vi "诊断标定3 - 副本.vi"(8 "CAN端口":u16(ring), 9 "设备索引号":u16(ring), 10 "CAN卡类型":u32(ring)=21) -> ()   [LabVIEW 2013] (continued)
                    }
                    frame True {
                      n418 = case shown="假" w611 {
                        tunnel: w618 -> [w622 _]
                        tunnel: w617 -> [w621 _]
                        tunnel: w616 -> [w620 _]
                        tunnel: w612 -> [w619 w846]
                        frame False {
                          n419 = case shown="89" w620 {
                            tunnel: w621 -> [_ w625]
                            tunnel: w622 -> [_ w624]
                            tunnel: w619 -> [_ _]
                            frame 0, Default {
                            }
                            frame 137 {
                              n420 = case shown="1" w625 {
                                tunnel: w624 -> [_ w653 w697 w717 w844]
                                frame 0, Default {
                                }
                                frame 1 {
                                w635 = "." ("字符串")
                                n421 = Array Subset(array=w653, index=0 ("索引"), length=14 ("长度")) -> (w666:u8[])
                                n422 = Index Array(array=w653, index=14 ("索引")) -> (element=w656:u8)
                                n423 = Index Array(array=w653, index #1=15 ("索引"), index #2=16 ("索引")) -> (element #1=w662:u8, element #2=w663:u8)
                                n424 = Index Array(array=w653, index #1=17 ("索引"), index #2=18 ("索引")) -> (element #1=w657:u8, element #2=w658:u8)
                                n425 = call "数组去零.vi"("输入"=w666) -> ("输出"=w641:dbl[])
                                n426 = Join Numbers(hi=w657, lo=w658) -> ((hi.lo)=w654:u16)
                                n427 = Join Numbers(hi=w662, lo=w663) -> ((hi.lo)=w655:u16)
                                n428 = Number To Decimal String(number=w656) -> (decimal integer string=w648:string)  [unwired: 1 out]
                                n429 = Byte Array To String(unsigned byte array=w641) -> (string=w640:string)
                                n430 = Number To Decimal String(number=w654) -> (decimal integer string=w636:string)  [unwired: 1 out]
                                n431 = Number To Decimal String(number=w655) -> (decimal integer string=w647:string)  [unwired: 1 out]
                                n432 = Array Subset(array=w653, index=21 ("索引"), length=7 ("长度")) -> (w650:u8[])
                                n433 = Concatenate Strings("V" ("字符串"), w648, w635, w647, w635, w636) -> (w645:string)
                                n434 = call "数组去零.vi"("输入"=w650) -> ("输出"=w633:dbl[])
                                n435 = Byte Array To String(unsigned byte array=w633) -> (string=w631:string)
                                n436 = call <vilib>:"Space Constant.vi"() -> ("String"=w632:string)
                                n437 = Equal?(x=w631, y=w632) -> (x = y?=w637:bool)
                                n438 = Concatenate Strings("-" ("字符串"), w631) -> (w638:string)
                                n439 = Select(t=w632, s=w637, f=w638) -> (s? t:f=w634:string)
                                n440 = Concatenate Strings(w640, "-" ("字符串"), w645, w634) -> (w627:string)
                                n441 = local read "项目软件版本"() -> (w629:string[])
                                n442 = local read "从板板号"() -> (w626:u8)
                                n443 = local write "项目软件版本号"(w627) -> ()
                                n444 = Replace Array Subset(array=w629, new element=w627, index=w626) -> (w628:string[])
                                n445 = control-ref of="结果"() -> (w644:refnum<vi>)
                                n446 = local write "项目软件版本"(w628) -> ()
                                n447 = Build Array("项目软件版本     读取完成" ("读取结果")) -> (w642:string[])
                                n448 = call "表格编辑(版本读取).vi"("新元素/子数组"=w642, "活动单元格:单元格背景色"=u32 6618880, "MCListbox引用句柄"=w644) -> ()  [unwired: 9 out]
                                }
                                frame 2 {
                                w680 = ""
                                w677 = "." ("字符串")
                                n449 = Array Subset(array=w697, index=0 ("索引"), length=14 ("长度")) -> (w685:u8[])
                                n450 = Index Array(array=w697, index=14 ("索引")) -> (element=w700:u8)
                                n451 = Index Array(array=w697, index #1=15 ("索引"), index #2=16 ("索引")) -> (element #1=w706:u8, element #2=w707:u8)
                                n452 = Index Array(array=w697, index #1=17 ("索引"), index #2=18 ("索引")) -> (element #1=w701:u8, element #2=w702:u8)
                                n453 = Join Numbers(hi=w701, lo=w702) -> ((hi.lo)=w698:u16)
                                n454 = Join Numbers(hi=w706, lo=w707) -> ((hi.lo)=w699:u16)
                                n455 = Number To Decimal String(number=w698) -> (decimal integer string=w678:string)  [unwired: 1 out]
                                n456 = call "数组去零.vi"("输入"=w685) -> ("输出"=w684:dbl[])
                                n457 = Number To Decimal String(number=w700) -> (decimal integer string=w692:string)  [unwired: 1 out]
                                n458 = Number To Decimal String(number=w699) -> (decimal integer string=w691:string)  [unwired: 1 out]
                                n459 = Array Subset(array=w697, index=21 ("索引"), length=7 ("长度")) -> (w694:u8[])
                                n460 = Byte Array To String(unsigned byte array=w684) -> (string=w679:string)
                                n461 = call "数组去零.vi"("输入"=w694) -> ("输出"=w676:dbl[])
                                n462 = Concatenate Strings("V" ("字符串"), w692, w677, w691, w677, w678) -> (w689:string)
                                n463 = Byte Array To String(unsigned byte array=w676) -> (string=w674:string)
                                n464 = Equal?(x=w680, y=w674) -> (x = y?=w681:bool)
                                n465 = Concatenate Strings("-" ("字符串"), w674) -> (w682:string)
                                n466 = Select(t=w680, s=w681, f=w682) -> (s? t:f=w675:string)
                                n467 = Concatenate Strings(w679, "-" ("字符串"), w689, w675) -> (w670:string)
                                n468 = local read "平台软件版本"() -> (w672:string[])
                                n469 = local read "从板板号"() -> (w669:u8)
                                n470 = local write "平台软件版本号"(w670) -> ()
                                n471 = Replace Array Subset(array=w672, new element=w670, index=w669) -> (w671:string[])
                                n472 = control-ref of="结果"() -> (w687:refnum<vi>)
                                n473 = local write "平台软件版本"(w671) -> ()
                                n474 = Build Array("平台软件版本     读取完成" ("读取结果")) -> (w686:string[])
                                n475 = call "表格编辑(版本读取).vi"("新元素/子数组"=w686, "活动单元格:单元格背景色"=u32 6618880, "MCListbox引用句柄"=w687) -> ()  [unwired: 1 in, 8 out]
                                }
                                frame 3 {
                                n476 = Index Array(array=w717, index #1=0 ("索引"), index #2=1 ("索引")) -> (element #1=w713:u8, element #2=w714:u8)
                                n477 = Join Numbers(hi=w713, lo=w714) -> ((hi.lo)=w712:u16)
                                n478 = case shown="99, 默认" w712 {
                                tunnel: w717 -> [w720 _ w754]
                                tunnel: w712 -> [_ _ w732]
                                frame 0 {
                                n479 = Index Array(array=w720, index #1=2 ("索引"), index #2=3 ("索引")) -> (element #1=w724:u8, element #2=w723:u8)
                                n480 = Join Numbers(hi=w724, lo=w723) -> ((hi.lo)=w719:u16)
                                n481 = for {
                                N: w719 -> [_]
                                tunnel: w720 -> [w729]
                                tunnel: [w725] -> w718 mode=indexing
                                i -> [w728]
                                n482 = Add(x=w728, y=4) -> (x+y=w726:i32)
                                n483 = Index Array(array=w729, index=w726) -> (element=w725:u8)
                                }
                                "MODEL号" <- w718
                                }
                                frame 99, Default {
                                }
                                frame 1..40 {
                                w737 = ""
                                w758 = "." ("字符串")
                                n484 = Array Subset(array=w754, index=2 ("索引"), length=14 ("长度")) -> (w743:u8[])
                                n485 = Index Array(array=w754, index=16 ("索引")) -> (element=w766:u8)
                                n486 = Index Array(array=w754, index #1=17 ("索引"), index #2=18 ("索引")) -> (element #1=w772:u8, element #2=w773:u8)
                                n487 = Index Array(array=w754, index #1=19 ("索引"), index #2=20 ("索引")) -> (element #1=w767:u8, element #2=w768:u8)
                                n488 = Join Numbers(hi=w767, lo=w768) -> ((hi.lo)=w764:u16)
                                n489 = Join Numbers(hi=w772, lo=w773) -> ((hi.lo)=w765:u16)
                                n490 = Number To Decimal String(number=w732) -> (decimal integer string=w752:string)  [unwired: 1 out]
                                n491 = Number To Decimal String(number=w766) -> (decimal integer string=w760:string)  [unwired: 1 out]
                                n492 = call "数组去零.vi"("输入"=w743) -> ("输出"=w742:dbl[])
                                n493 = Number To Decimal String(number=w765) -> (decimal integer string=w759:string)  [unwired: 1 out]
                                n494 = Number To Decimal String(number=w764) -> (decimal integer string=w757:string)  [unwired: 1 out]
                                n495 = Byte Array To String(unsigned byte array=w742) -> (string=w744:string)
                                n496 = Concatenate Strings("第" ("读取结果"), w752, "模块" ("字符串"), "     读取完成" ("读取结果")) -> (w745:string)
                                n497 = Concatenate Strings("V" ("字符串"), w760, w758, w759, w758, w757) -> (w755:string)
                                n498 = control-ref of="结果"() -> (w748:refnum<vi>)
                                n499 = Array Subset(array=w754, index=23 ("索引"), length=7 ("长度")) -> (w741:u8[])
                                n500 = call "数组去零.vi"("输入"=w741) -> ("输出"=w736:dbl[])
                                n501 = Byte Array To String(unsigned byte array=w736) -> (string=w733:string)
                                n502 = Build Array(w745) -> (w747:string[])
                                n503 = control-ref of="模块软件版本 2"() -> (w749:refnum<vi>)
                                n504 = local read "模块软件版本"() -> (w750:T1)
                                n505 = Equal?(x=w737, y=w733) -> (x = y?=w738:bool)
                                n506 = call "表格编辑(版本读取).vi"("新元素/子数组"=w747, "活动单元格:单元格背景色"=u32 6618880, "MCListbox引用句柄"=w748) -> ()  [unwired: 1 in, 8 out]
                                n507 = Concatenate Strings("-" ("字符串"), w733) -> (w739:string)
                                n508 = Select(t=w737, s=w738, f=w739) -> (s? t:f=w735:string)
                                n509 = Concatenate Strings(w744, "-" ("字符串"), w755, w735) -> (w734:string)
                                n510 = case shown="30" w732 {
                                tunnel: [_ "VERSIONM" "BCUMCAL" "BMUMCAL" "BMURMCAL" "BCUCMCAL" "BCUDMCAL" "SCH" "BSW" "CDD" "DATALAYER" "DATAANALYSIS" "SOC" "SOH" "SOF" "INTRES" "INTCAN" "CARCAN" "CHGCANL" "THM" "CHGM" "HVM" "LVM" "BALM" "SAFEM" "RUNMODEM" "RELAY" "DO" "GBCHGDET" "SUPPLYPOWGDET" "SUMVDET" "CURDET" "TEMPERDET" "CELLVDET" "ISODET" "AI" "DI" "SYSCONF" "ECUCONF"] -> w731
                                frame 0, Default {
                                }
                                frame 1 {
                                }
                                frame 2 {
                                }
                                frame 3 {
                                }
                                frame 4 {
                                }
                                frame 5 {
                                }
                                frame 6 {
                                }
                                frame 7 {
                                }
                                frame 8 {
                                }
                                frame 9 {
                                }
                                frame 10 {
                                }
                                frame 11 {
                                }
                                frame 12 {
                                }
                                frame 13 {
                                }
                                frame 14 {
                                }
                                frame 15 {
                                }
                                frame 16 {
                                }
                                frame 17 {
                                }
                                frame 18 {
                                }
                                frame 19 {
                                }
                                frame 20 {
                                }
                                frame 21 {
                                }
                                frame 22 {
                                }
                                frame 23 {
                                }
                                frame 24 {
                                }
                                frame 25 {
                                }
                                frame 26 {
                                }
                                frame 27 {
                                }
                                frame 28 {
                                }
                                frame 29 {
                                }
                                frame 30 {
                                }
                                frame 31 {
                                }
                                frame 32 {
                                }
                                frame 33 {
                                }
                                frame 34 {
                                }
                                frame 35 {
                                }
                                frame 36 {
                                }
                                frame 37 {
                                }
                                frame 38 {
                                }
                                }
                                n511 = case shown="\"全部读取\"" w750 {
                                tunnel: w734 -> [w817 w825]
                                tunnel: w732 -> [w821 w830]
                                tunnel: w749 -> [w823 w831]
                                tunnel: w731 -> [w822 w829]
                                frame "全部读取" {
                                n512 = Number To Decimal String(number=w821) -> (decimal integer string=w820:string)  [unwired: 1 out]
                                n513 = Concatenate Strings(w820, "-" ("元素"), w822) -> (w818:string)
                                n514 = Build Array(w818, w817) -> (w816:string[])
                                n515 = call "表格编辑(模块版本).vi"("新元素/子数组"=w816, "MCListbox引用句柄"=w823) -> ()  [unwired: 1 in, 9 out]
                                }
                                frame "BCUMCAL", Default {
                                n516 = Number To Decimal String(number=w830) -> (decimal integer string=w828:string)  [unwired: 1 out]
                                n517 = Concatenate Strings(w828, "-" ("元素"), w829) -> (w826:string)
                                n518 = Build Array(w826, w825) -> (w824:string[])
                                n519 = call "表格编辑(模块版本).vi"("新元素/子数组"=w824, "MCListbox引用句柄"=w831) -> ()  [unwired: 1 in, 9 out]
                                }
                                }
                                }
                                }
                                }
                                frame 4 {
                                n520 = Array Subset(array=w844, length=12 ("长度")) -> (w842:u8[])  [unwired: 1 in]
                                n521 = Byte Array To String(unsigned byte array=w842) -> (string=w841:string)
                                n522 = call <vilib>:"Trim Whitespace.vi"("string"=w841) -> ("trimmed string"=w833:string)  [unwired: 1 in]
                                n523 = local read "从板板号"() -> (w832:u8)
                                n524 = local write "硬件版本号"(w833) -> ()
                                n525 = local read "硬件版本"() -> (w834:string[])
                                n526 = Replace Array Subset(array=w834, new element=w833, index=w832) -> (w835:string[])
                                n527 = local write "硬件版本"(w835) -> ()
                                n528 = global write "EV05全局变量1.vi" "写入超时"(TRUE ("写入超时")) -> ()
                                n529 = control-ref of="结果"() -> (w839:refnum<vi>)
                                n530 = Build Array("硬件版本     读取完成" ("读取结果")) -> (w838:string[])
                                n531 = call "表格编辑(版本读取).vi"("新元素/子数组"=w838, "活动单元格:单元格背景色"=u32 6618880, "MCListbox引用句柄"=w839) -> ()  [unwired: 9 out]
                                }
                              }
                              n532 = global write "EV05全局变量1.vi" "写入超时"(TRUE ("写入超时")) -> ()
                            }
                          }
                        }
                        frame True {
                          n533 = Index Array(array=w846, index #1=0 ("索引"), index #2=1 ("索引")) -> (element #1=w851:u8, element #2=w852:u8)
                          n534 = Join Numbers(hi=w851, lo=w852) -> ((hi.lo)=w850:u16)
                          n535 = Number To Hexadecimal String(2:w850) -> (0:w849:string)  [unwired: 1 out]
                          n536 = control-ref of="结果"() -> (w848:refnum<vi>)
                          n537 = Concatenate Strings("0x" ("字符串"), w849) -> (w856:string)
                          n538 = Build Array(w856) -> (w847:string[])
                          n539 = call "表格编辑(版本读取).vi"("新元素/子数组"=w847, "活动单元格:单元格背景色"=u32 16740749, "MCListbox引用句柄"=w848) -> ()  [unwired: 9 out]
                        }
                      }
                      n540 = global write "EV05全局变量1.vi" "流控帧 2"(FALSE ("流控帧 2")) -> ()
                      n541 = local write "控制1"(FALSE ("控制1")) -> ()
                      n542 = local write "消除"(FALSE ("消除")) -> ()
                      n543 = call <vilib>:"Unset Busy.vi"() -> ()  [unwired: 2 in, 10 out]
                    }
                  }
                }
                frame "其它诊断" {
                  n544 = local read "命令序号"() -> (w858:u8)
                  n545 = call "多帧接收机制(EV05).vi"("can卡类型"=w865, "设备索引号"=w864, "CAN端口"=w863, "VCI_Receive"=w862, "命令"=w860, "板号"=w861, "命令序号"=w858) -> ("错误代码"=w867:i32, "输出数组"=w859:u8[], "读错误代码"=w857:u8[], "结束信号"=w866:bool)  [unwired: 1 in, 8 out]
                  n546 = case shown="真" w866 {
                    tunnel: w868 -> [_ w869]
                    tunnel: w867 -> [_ _]
                    tunnel: w859 -> [_ w870]
                    tunnel: w858 -> [_ w873]
                    tunnel: w857 -> [_ w871]
                    frame False {
                    }
                    frame True {
                      n547 = Insert Into Array(array=w871, new element=w870) -> (w872:u8[])  [unwired: 1 in]
                      n548 = case shown="1" w873 {
                        tunnel: w872 -> [_ w882 w968]
                        tunnel: w869 -> [_ _ w963]
                        frame 0, Default {
                        }
                        frame 1 {
                          n549 = Index Array(array=w882) -> (element #1=w881:u8, element #2=w880:u8, element #3=w879:u8)  [unwired: 3 in]
                          n550 = Join Numbers(hi=w880, lo=w879) -> ((hi.lo)=w878:u16)
                          n551 = case shown="4" w881 {
                            tunnel: w882 -> [_ _ _ _ _ _ _ _ _ _]
                            tunnel: w878 -> [_ w885 w893 w903 w913 w923 w933 w943 w953 _]
                            frame 0, Default {
                              n552 = local write "继电器超时处理"(FALSE ("继电器超时处理")) -> ()
                            }
                            frame 1 {
                              n553 = Equal To 0?(x=w885) -> (x = 0?=w884:bool)
                              n554 = local write "正级继电器 12"(w884) -> ()
                              n555 = case shown="假" w884 {
                                tunnel: w885 -> [w888 _]
                                frame False {
                                n556 = local read "正级继电器"() -> (w890:bool)
                                n557 = Number To Hexadecimal String(2:w888) -> (0:w887:string)  [unwired: 1 out]
                                n558 = local write "继电器超时处理"(TRUE ("继电器超时处理")) -> ()
                                n559 = Not(x=w890) -> (.not. x?=w889:bool)
                                n560 = Concatenate Strings("继电器操作失败,0x" ("消息"), w887) -> ()  [unwired: 1 out]
                                n561 = local write "正级继电器"(w889) -> ()
                                }
                                frame True {
                                (unwired) "继电器操作成功!\n继电器操作成功!\n继电器操作成功!"
                                }
                              }
                            }
                            frame 2 {
                              n562 = Equal To 0?(x=w893) -> (x = 0?=w892:bool)
                              n563 = case shown="假" w892 {
                                tunnel: w893 -> [w899 _]
                                tunnel: [w897 "继电器操作成功!\n继电器操作成功!\n继电器操作成功!"] -> _
                                frame False {
                                n564 = local read "负级继电器"() -> (w895:bool)
                                n565 = Number To Hexadecimal String(2:w899) -> (0:w898:string)  [unwired: 1 out]
                                n566 = local write "继电器超时处理"(TRUE ("继电器超时处理")) -> ()
                                n567 = Not(x=w895) -> (.not. x?=w896:bool)
                                n568 = Concatenate Strings("继电器操作失败,0x" ("消息"), w898) -> (w897:string)
                                n569 = local write "负级继电器"(w896) -> ()
                                }
                                frame True {
                                }
                              }
                              n570 = local write "正级继电器 2"(w892) -> ()
                            }
                            frame 3 {
                              n571 = Equal To 0?(x=w903) -> (x = 0?=w902:bool)
                              n572 = case shown="假" w902 {
                                tunnel: w903 -> [w909 _]
                                tunnel: [w907 "继电器操作成功!\n继电器操作成功!\n继电器操作成功!"] -> _
                                frame False {
                                n573 = local read "预充电继电器"() -> (w905:bool)
                                n574 = Number To Hexadecimal String(2:w909) -> (0:w908:string)  [unwired: 1 out]
                                n575 = local write "继电器超时处理"(TRUE ("继电器超时处理")) -> ()
                                n576 = Not(x=w905) -> (.not. x?=w906:bool)
                                n577 = Concatenate Strings("继电器操作失败,0x" ("消息"), w908) -> (w907:string)
                                n578 = local write "预充电继电器"(w906) -> ()
                                }
                                frame True {
                                }
                              }
                              n579 = local write "正级继电器 3"(w902) -> ()
                            }
                            frame 4 {
                              n580 = Equal To 0?(x=w913) -> (x = 0?=w912:bool)
                              n581 = case shown="假" w912 {
                                tunnel: w913 -> [w919 _]
                                tunnel: [w917 "继电器操作成功!\n继电器操作成功!\n继电器操作成功!"] -> _
                                frame False {
                                n582 = local read "加热继电器"() -> (w916:bool)
                                n583 = Number To Hexadecimal String(2:w919) -> (0:w918:string)  [unwired: 1 out]
                                n584 = local write "继电器超时处理"(TRUE ("继电器超时处理")) -> ()
                                n585 = Not(x=w916) -> (.not. x?=w915:bool)
                                n586 = Concatenate Strings("继电器操作失败,0x" ("消息"), w918) -> (w917:string)
                                n587 = local write "加热继电器"(w915) -> ()
                                }
                                frame True {
                                }
                              }
                              n588 = local write "正级继电器 5"(w912) -> ()
                            }
                            frame 5 {
                              n589 = Equal To 0?(x=w923) -> (x = 0?=w922:bool)
                              n590 = case shown="假" w922 {
                                tunnel: w923 -> [w929 _]
                                tunnel: [w927 "继电器操作成功!\n继电器操作成功!\n继电器操作成功!"] -> _
                                frame False {
                                n591 = local read "充电继电器"() -> (w925:bool)
                                n592 = Number To Hexadecimal String(2:w929) -> (0:w928:string)  [unwired: 1 out]
                                n593 = local write "继电器超时处理"(TRUE ("继电器超时处理")) -> ()
                                n594 = Not(x=w925) -> (.not. x?=w926:bool)
                                n595 = Concatenate Strings("继电器操作失败,0x" ("消息"), w928) -> (w927:string)
                                n596 = local write "充电继电器"(w926) -> ()
                                }
                                frame True {
                                }
                              }
                              n597 = local write "正级继电器 4"(w922) -> ()
                            }
                            frame 6 {
                              n598 = Equal To 0?(x=w933) -> (x = 0?=w932:bool)
                              n599 = local write "正级继电器 6"(w932) -> ()
                              n600 = case shown="假" w932 {
                                tunnel: w933 -> [w939 _]
                                tunnel: [w937 "继电器操作成功!\n继电器操作成功!\n继电器操作成功!"] -> _
                                frame False {
                                n601 = local read "风机继电器"() -> (w935:bool)
                                n602 = Number To Hexadecimal String(2:w939) -> (0:w938:string)  [unwired: 1 out]
                                n603 = local write "继电器超时处理"(TRUE ("继电器超时处理")) -> ()
                                n604 = Not(x=w935) -> (.not. x?=w936:bool)
                                n605 = Concatenate Strings("继电器操作失败,0x" ("消息"), w938) -> (w937:string)
                                n606 = local write "风机继电器"(w936) -> ()
                                }
                                frame True {
                                }
                              }
                            }
                            frame 7 {
                              n607 = Equal To 0?(x=w943) -> (x = 0?=w942:bool)
                              n608 = case shown="假" w942 {
                                tunnel: w943 -> [w948 _]
                                tunnel: [w946 "继电器操作成功!\n继电器操作成功!\n继电器操作成功!"] -> _
                                frame False {
                                n609 = local read "加热继电器(从)"() -> (w944:bool)
                                n610 = Number To Hexadecimal String(2:w948) -> (0:w947:string)  [unwired: 1 out]
                                n611 = Not(x=w944) -> (.not. x?=w945:bool)
                                n612 = Concatenate Strings("继电器操作失败,0x" ("消息"), w947) -> (w946:string)
                                n613 = local write "加热继电器(从)"(w945) -> ()
                                }
                                frame True {
                                n614 = local write "继电器超时处理"(TRUE ("继电器超时处理")) -> ()
                                }
                              }
                              n615 = local write "正级继电器 7"(w942) -> ()
                            }
                            frame 8 {
                              n616 = Equal To 0?(x=w953) -> (x = 0?=w952:bool)
                              n617 = case shown="假" w952 {
                                tunnel: w953 -> [w958 _]
                                tunnel: [w956 "继电器操作成功!\n继电器操作成功!\n继电器操作成功!"] -> _
                                frame False {
                                n618 = local read "风机继电器(从)"() -> (w954:bool)
                                n619 = Number To Hexadecimal String(2:w958) -> (0:w957:string)  [unwired: 1 out]
                                n620 = Not(x=w954) -> (.not. x?=w955:bool)
                                n621 = Concatenate Strings("继电器操作失败,0x" ("消息"), w957) -> (w956:string)
                                n622 = local write "风机继电器(从)"(w955) -> ()
                                }
                                frame True {
                                n623 = local write "继电器超时处理"(TRUE ("继电器超时处理")) -> ()
                                }
                              }
                              n624 = local write "正级继电器 8"(w952) -> ()
                            }
                            frame 85, 170 {
                              n625 = local write "继电器超时处理"(TRUE ("继电器超时处理")) -> ()
                            }
                          }
                        }
                        frame 2 {
                          n626 = Index Array(array=w968) -> (element #1=w967:u8, element #2=w966:u8, element #3=w965:u8)  [unwired: 3 in]
                          n627 = Join Numbers(hi=w966, lo=w965) -> ((hi.lo)=w964:u16)
                          n628 = case shown="2" w967 {
                            tunnel: w968 -> [_ _ _]
                            tunnel: w964 -> [_ w972 w986]
                            tunnel: w963 -> [_ w971 _]
                            frame 0, Default {
                              n629 = local write "继电器超时处理"(FALSE ("继电器超时处理")) -> ()
                            }
                            frame 1 {
                              n630 = Equal To 0?(x=w972) -> (x = 0?=w970:bool)
                              n631 = case shown="假" w970 {
                                tunnel: w972 -> [w978 _]
                                tunnel: [w976 "DO控制操作成功!\nDO控制操作成功!\nDO控制操作成功!"] -> _
                                tunnel: w971 -> [w975 _]
                                frame False {
                                n632 = case shown="\"主板\", 默认" w975 {
                                frame "主板", Default {
                                n633 = local read "DO1"() -> (w981:bool)
                                n634 = Not(x=w981) -> (.not. x?=w980:bool)
                                n635 = local write "DO1"(w980) -> ()
                                }
                                frame "从板" {
                                n636 = local read "DO1 2"() -> (w983:bool)
                                n637 = Not(x=w983) -> (.not. x?=w982:bool)
                                n638 = local write "DO1 2"(w982) -> ()
                                }
                                }
                                n639 = Number To Hexadecimal String(2:w978) -> (0:w977:string)  [unwired: 1 out]
                                n640 = Concatenate Strings("DO控制操作失败,0x" ("消息"), w977) -> (w976:string)
                                }
                                frame True {
                                }
                              }
                              n641 = case shown="\"从板\"" w971 {
                                tunnel: w970 -> [w973 w974]
                                frame "主板", Default {
                                n642 = local write "正级继电器 9"(w973) -> ()
                                }
                                frame "从板" {
                                n643 = local write "正级继电器 11"(w974) -> ()
                                }
                              }
                            }
                            frame 2 {
                              n644 = Equal To 0?(x=w986) -> (x = 0?=w985:bool)
                              n645 = case shown="假" w985 {
                                tunnel: w986 -> [w991 _]
                                tunnel: [w989 "DO控制操作成功!\nDO控制操作成功!\nDO控制操作成功!"] -> _
                                frame False {
                                n646 = Number To Hexadecimal String(2:w991) -> (0:w990:string)  [unwired: 1 out]
                                n647 = local read "DO2"() -> (w988:bool)
                                n648 = Not(x=w988) -> (.not. x?=w987:bool)
                                n649 = Concatenate Strings("DO控制操作失败,0x" ("消息"), w990) -> (w989:string)
                                n650 = local write "DO2"(w987) -> ()
                                }
                                frame True {
                                }
                              }
                              n651 = local write "正级继电器 10"(w985) -> ()
                            }
                          }
                        }
                      }
                      n652 = local write "消除"(FALSE ("消除")) -> ()
                      n653 = global write "EV05全局变量1.vi" "流控帧 2"(FALSE ("流控帧 2")) -> ()
                      n654 = local write "控制1"(FALSE ("控制1")) -> ()
                      "继电器超时处理" <- TRUE ("控制1")
                    }
                  }
                }
                frame "高压板校正" {
                  n655 = local read "命令序号"() -> (w998:u8)
                  n656 = call "多帧接收机制(EV05).vi"("can卡类型"=w1005, "设备索引号"=w1004, "CAN端口"=w1003, "VCI_Receive"=w1002, "命令"=w1000, "板号"=w1001, "命令序号"=w998) -> ("错误信号"=w994:bool, "错误代码"=w1007:i32, "输出数组"=w999:u8[], "读错误代码"=w997:u8[], "结束信号"=w1006:bool)  [unwired: 1 in, 7 out]
                  n657 = local read "控制1"() -> (w995:bool)
                  n658 = And(x=w995, y=w1006) -> (x .and. y?=w996:bool)
                  n659 = case shown="真" w996 {
                    tunnel: w1008 -> [_ w1012]
                    tunnel: w1007 -> [_ _]
                    tunnel: w999 -> [_ w1010]
                    tunnel: w998 -> [_ w1011]
                    tunnel: w997 -> [_ w1013]
                    tunnel: w994 -> [_ w1014]
                    frame False {
                    }
                    frame True {
                      n660 = case shown="假" w1014 {
                        tunnel: w1013 -> [_ w1224]
                        tunnel: w1012 -> [_ _]
                        tunnel: w1011 -> [w1019 _]
                        tunnel: w1010 -> [w1018 _]
                        frame False {
                          n661 = case shown="2" w1019 {
                            tunnel: w1018 -> [_ w1024 w1058 w1088 w1115 w1142 w1169 w1196]
                            frame 0, Default {
                            }
                            frame 1 {
                              n662 = for {
                                N: 10 -> [_]
                                tunnel: w1024 -> [w1041]
                                shift-right: [w1028] -> w1022
                                shift-left: string[] [] -> [w1030]
                                i -> [w1027]
                                w1035 = 8 ("索引")
                                w1039 = 2 ("y")
                                n663 = Multiply(x=w1027, y=w1039) -> (x*y=w1040:i32)
                                n664 = Array Subset(array=w1041, index=w1040, length=w1039) -> (w1038:u8[])
                                n665 = Index Array(array=w1038) -> (element #1=w1037:u8, element #2=w1036:u8)  [unwired: 2 in]
                                n666 = call "二进制解析-8.6.vi"("索引"=w1035, "数值"=w1037) -> ("低位子数组"=w1034:i32[])  [unwired: 1 in, 2 out]
                                n667 = call "二进制解析-8.6.vi"("索引"=w1035, "数值"=w1036) -> ("低位子数组"=w1033:i32[])  [unwired: 1 in, 2 out]
                                n668 = Insert Into Array(array=w1034, new element=w1033) -> (w1032:i32[])  [unwired: 1 in]
                                n669 = case shown="2" w1027 {
                                tunnel: [6 15 9 4 2 0 2] -> w1026
                                frame 0, Default {
                                }
                                frame 1 {
                                }
                                frame 2 {
                                }
                                frame 3..5 {
                                }
                                frame 8, 9 {
                                }
                                frame 7 {
                                }
                                frame 6 {
                                }
                                }
                                n670 = Reverse 1D Array(array=w1032) -> (reversed array=w1031:i32[])
                                n671 = for {
                                N: w1026 -> [_]
                                tunnel: w1031 -> [w1053] mode=indexing
                                tunnel: [w1049] -> w1029 mode=indexing
                                n672 = Equal To 0?(x=w1053) -> (x = 0?=w1052:bool)
                                n673 = Select(t="无", s=w1052, f="故障") -> (s? t:f=w1049:string)
                                }
                                n674 = Insert Into Array(array=w1030, new element=w1029) -> (w1028:string[])  [unwired: 1 in]
                              }
                              n675 = call "详细故障分解.vi"("名称"=string[] ["上电自检异常(CellV)", "通讯异常(CellV)", "不更新(CellV)", "未校准(CellV)", "保留", "采样线路断路(CellV)", "18b20上电自检异常(T) ", "18b20通讯异常(T)", "18b20传感器丢失(T)", "18b20传感器无号(T)", "18b20温度异常跳变(T)", "18b20信号线对电源短路(T)", "18b20信号线对地短路(T)", "18b20 CRC校验异常(T)", "NTC上电自检异常(T)", "NTC通讯异常(T)", "NTC传感器丢失(T)", "NTC温度异常跳变(T)", "NTC信号线断路(T)", "NTC信号线对电源短(T)", "NTC信号线对地短路(T)", "上电自检异常(Curr)", "参数异常(Curr)", "不更新(Curr)", "未校准(Curr)", "采样线断开(Curr)", "电流零漂异常(Curr)", "传感器反接(Curr)", "读取实时电流故障(Curr)", "平均电流故障(Curr)", "自检异常(iso)", "前端检测电阻损坏(iso)", "不更新(iso)", "未校准(iso)", "上电自检异常(Sumv_in)", "通讯异常(Sumv_in)", "不更新(Sumv_in)", "未校准(Sumv_in)", "上电自检异常(Sumv_out)", "通讯异常(Sumv_out)", "不更新(Sumv_out)", "未校准(Sumv_out)", "系统时钟自检异常(Clock)", "系统时钟未校准(Clock)", "充电均衡模块不能开启", "充电均衡模块不能关闭", "放电均衡模块不能开启", "放电均衡模块不能关闭"], "故障输入口"=w1022) -> ("输出数组"=w1020:string[][])  [unwired: 1 in, 2 out]
                              n676 = local write "电池故障"(w1020) -> ()
                            }
                            frame 2 {
                              n677 = for {
                                N: 5 -> [_]
                                tunnel: w1058 -> [w1075]
                                shift-right: [w1062] -> w1056
                                shift-left: string[] [] -> [w1064]
                                i -> [w1060]
                                w1069 = 8 ("索引")
                                w1073 = 2 ("y")
                                n678 = Multiply(x=w1060, y=w1073) -> (x*y=w1074:i32)
                                n679 = Array Subset(array=w1075, index=w1074, length=w1073) -> (w1072:u8[])
                                n680 = Index Array(array=w1072) -> (element #1=w1071:u8, element #2=w1070:u8)  [unwired: 2 in]
                                n681 = call "二进制解析-8.6.vi"("索引"=w1069, "数值"=w1071) -> ("低位子数组"=w1068:i32[])  [unwired: 1 in, 2 out]
                                n682 = call "二进制解析-8.6.vi"("索引"=w1069, "数值"=w1070) -> ("低位子数组"=w1067:i32[])  [unwired: 1 in, 2 out]
                                n683 = Insert Into Array(array=w1068, new element=w1067) -> (w1066:i32[])  [unwired: 1 in]
                                n684 = case shown="2" w1060 {
                                tunnel: [4 6 5] -> w1061
                                frame 0, Default {
                                }
                                frame 2 {
                                }
                                frame 4 {
                                }
                                }
                                n685 = Reverse 1D Array(array=w1066) -> (reversed array=w1065:i32[])
                                n686 = for {
                                N: w1061 -> [_]
                                tunnel: w1065 -> [w1083] mode=indexing
                                tunnel: [w1079] -> w1063 mode=indexing
                                n687 = Equal To 0?(x=w1083) -> (x = 0?=w1082:bool)
                                n688 = Select(t="无", s=w1082, f="故障") -> (s? t:f=w1079:string)
                                }
                                n689 = Insert Into Array(array=w1064, new element=w1063) -> (w1062:string[])  [unwired: 1 in]
                              }
                              n690 = call "详细故障分解.vi"("名称"=string[] ["自检异常(ee_cpu)", "存储空间满(ee_cpu)", "数据写入失败(ee_cpu)", "数据读取异常(ee_cpu)", "自检异常(ee_ext)", "存储空间满(ee_ext)", "数据写入失败(ee_ext)", "数据读取异常(ee_ext)", "自检异常(flash_ext)", "故障数据存储空间满(flash_ext)", "历史数据存储空间满(flash_ext)", "数据写入失败(flash_ext)", "数据读取失败(flash_ext)", "数据校验异常(flash_ext)", "自检异常(flash_cpu)", "存储空间满(flash_cpu)", "数据写入失败(flash_cpu)", "数据读取异常(flash_cpu)", "应用程序异常(cpu)", "应用程序下载异常(cpu)", "AD模块异常(cpu)", "RAM异常(cpu)", "CPU异常下电(cpu)"], "故障输入口"=w1056) -> ("输出数组"=w1054:string[][])  [unwired: 1 in, 2 out]
                              n691 = local write "电池故障"(w1054) -> ()
                            }
                            frame 3 {
                              n692 = for {
                                N: 5 -> [_]
                                tunnel: w1088 -> [w1105]
                                shift-right: [w1092] -> w1086
                                shift-left: string[] [] -> [w1094]
                                i -> [w1091]
                                w1099 = 8 ("索引")
                                w1103 = 2 ("y")
                                n693 = Multiply(x=w1091, y=w1103) -> (x*y=w1104:i32)
                                n694 = Array Subset(array=w1105, index=w1104, length=w1103) -> (w1102:u8[])
                                n695 = Index Array(array=w1102) -> (element #1=w1101:u8, element #2=w1100:u8)  [unwired: 2 in]
                                n696 = call "二进制解析-8.6.vi"("索引"=w1099, "数值"=w1101) -> ("低位子数组"=w1098:i32[])  [unwired: 1 in, 2 out]
                                n697 = call "二进制解析-8.6.vi"("索引"=w1099, "数值"=w1100) -> ("低位子数组"=w1097:i32[])  [unwired: 1 in, 2 out]
                                n698 = Insert Into Array(array=w1098, new element=w1097) -> (w1096:i32[])  [unwired: 1 in]
                                n699 = Reverse 1D Array(array=w1096) -> (reversed array=w1095:i32[])
                                n700 = for {
                                N: 6 -> [_]
                                tunnel: w1095 -> [w1110] mode=indexing
                                tunnel: [w1106] -> w1093 mode=indexing
                                n701 = Equal To 0?(x=w1110) -> (x = 0?=w1109:bool)
                                n702 = Select(t="无", s=w1109, f="故障") -> (s? t:f=w1106:string)
                                }
                                n703 = Insert Into Array(array=w1094, new element=w1093) -> (w1092:string[])  [unwired: 1 in]
                              }
                              n704 = call "详细故障分解.vi"("名称"=string[] ["初始化失败(CAN4)", "发送异常(CAN4)", "接收异常(CAN4)", "总线超时(CAN4)", "BUSOFF(CAN4)", "帧格式(CAN4)", "初始化异常(CAN0)", "发送异常(CAN0)", "接收异常(CAN0)", "总线超时(CAN0)", "BUSOFF(CAN0)", "帧格式(CAN0)", "初始化异常(CAN1)", "发送异常(CAN1)", "接收异常(CAN1)", "总线超时(CAN1)", "BUSOFF(CAN1)", "帧格式(CAN1)", "初始化失败(CAN2)", "发送异常(CAN2)", "接收异常(CAN2)", "总线超时(CAN2)", "BUSOFF(CAN2)", "帧格式(CAN2)", "初始化失败(CAN3)", "发送异常(CAN3)", "接收异常(CAN3)", "总线超时(CAN3)", "BUSOFF(CAN3)", "帧格式(CAN3)"], "故障输入口"=w1086) -> ("输出数组"=w1084:string[][])  [unwired: 1 in, 2 out]
                              n705 = local write "电池故障"(w1084) -> ()
                            }
                            frame 4 {
                              n706 = for {
                                N: 1 -> [_]
                                tunnel: w1115 -> [w1132]
                                shift-right: [w1119] -> w1113
                                shift-left: string[] [] -> [w1121]
                                i -> [w1118]
                                w1126 = 8 ("索引")
                                w1130 = 2 ("y")
                                n707 = Multiply(x=w1118, y=w1130) -> (x*y=w1131:i32)
                                n708 = Array Subset(array=w1132, index=w1131, length=w1130) -> (w1129:u8[])
                                n709 = Index Array(array=w1129) -> (element #1=w1128:u8, element #2=w1127:u8)  [unwired: 2 in]
                                n710 = call "二进制解析-8.6.vi"("索引"=w1126, "数值"=w1128) -> ("低位子数组"=w1125:i32[])  [unwired: 1 in, 2 out]
                                n711 = call "二进制解析-8.6.vi"("索引"=w1126, "数值"=w1127) -> ("低位子数组"=w1124:i32[])  [unwired: 1 in, 2 out]
                                n712 = Insert Into Array(array=w1125, new element=w1124) -> (w1123:i32[])  [unwired: 1 in]
                                n713 = Reverse 1D Array(array=w1123) -> (reversed array=w1122:i32[])
                                n714 = for {
                                N: 4 -> [_]
                                tunnel: w1122 -> [w1137] mode=indexing
                                tunnel: [w1133] -> w1120 mode=indexing
                                n715 = Equal To 0?(x=w1137) -> (x = 0?=w1136:bool)
                                n716 = Select(t="无", s=w1136, f="故障") -> (s? t:f=w1133:string)
                                }
                                n717 = Insert Into Array(array=w1121, new element=w1120) -> (w1119:string[])  [unwired: 1 in]
                              }
                              n718 = call "详细故障分解.vi"("名称"=string[] ["通讯协议版本不一致(soft)", "系统不同步(soft)", "软件版本不一致(soft)", "同硬件平台不兼容(soft)"], "故障输入口"=w1113) -> ("输出数组"=w1111:string[][])  [unwired: 1 in, 2 out]
                              n719 = local write "电池故障"(w1111) -> ()
                            }
                            frame 5 {
                              n720 = for {
                                N: 2 -> [_]
                                tunnel: w1142 -> [w1159]
                                shift-right: [w1146] -> w1140
                                shift-left: string[] [] -> [w1148]
                                i -> [w1145]
                                w1153 = 8 ("索引")
                                w1157 = 2 ("y")
                                n721 = Multiply(x=w1145, y=w1157) -> (x*y=w1158:i32)
                                n722 = Array Subset(array=w1159, index=w1158, length=w1157) -> (w1156:u8[])
                                n723 = Index Array(array=w1156) -> (element #1=w1155:u8, element #2=w1154:u8)  [unwired: 2 in]
                                n724 = call "二进制解析-8.6.vi"("索引"=w1153, "数值"=w1155) -> ("低位子数组"=w1152:i32[])  [unwired: 1 in, 2 out]
                                n725 = call "二进制解析-8.6.vi"("索引"=w1153, "数值"=w1154) -> ("低位子数组"=w1151:i32[])  [unwired: 1 in, 2 out]
                                n726 = Insert Into Array(array=w1152, new element=w1151) -> (w1150:i32[])  [unwired: 1 in]
                                n727 = Reverse 1D Array(array=w1150) -> (reversed array=w1149:i32[])
                                n728 = for {
                                N: 4 -> [_]
                                tunnel: w1149 -> [w1164] mode=indexing
                                tunnel: [w1160] -> w1147 mode=indexing
                                n729 = Equal To 0?(x=w1164) -> (x = 0?=w1163:bool)
                                n730 = Select(t="无", s=w1163, f="故障") -> (s? t:f=w1160:string)
                                }
                                n731 = Insert Into Array(array=w1148, new element=w1147) -> (w1146:string[])  [unwired: 1 in]
                              }
                              n732 = call "详细故障分解.vi"("名称"=string[] ["初始化失败(RS232)", "发送异常(RS232)", "接收异常(RS232)", "总线超时(RS232)", "初始化失败(RS485)", "发送异常(RS485)", "接收异常(RS485)", "总线超时(RS485)"], "故障输入口"=w1140) -> ("输出数组"=w1138:string[][])  [unwired: 1 in, 2 out]
                              n733 = local write "电池故障"(w1138) -> ()
                            }
                            frame 6 {
                              n734 = for {
                                N: 2 -> [_]
                                tunnel: w1169 -> [w1186]
                                shift-right: [w1173] -> w1167
                                shift-left: string[] [] -> [w1175]
                                i -> [w1172]
                                w1180 = 8 ("索引")
                                w1184 = 2 ("y")
                                n735 = Multiply(x=w1172, y=w1184) -> (x*y=w1185:i32)
                                n736 = Array Subset(array=w1186, index=w1185, length=w1184) -> (w1183:u8[])
                                n737 = Index Array(array=w1183) -> (element #1=w1182:u8, element #2=w1181:u8)  [unwired: 2 in]
                                n738 = call "二进制解析-8.6.vi"("索引"=w1180, "数值"=w1182) -> ("低位子数组"=w1179:i32[])  [unwired: 1 in, 2 out]
                                n739 = call "二进制解析-8.6.vi"("索引"=w1180, "数值"=w1181) -> ("低位子数组"=w1178:i32[])  [unwired: 1 in, 2 out]
                                n740 = Insert Into Array(array=w1179, new element=w1178) -> (w1177:i32[])  [unwired: 1 in]
                                n741 = Reverse 1D Array(array=w1177) -> (reversed array=w1176:i32[])
                                n742 = for {
                                N: 16 -> [_]
                                tunnel: w1176 -> [w1191] mode=indexing
                                tunnel: [w1187] -> w1174 mode=indexing
                                n743 = Equal To 0?(x=w1191) -> (x = 0?=w1190:bool)
                                n744 = Select(t="无", s=w1190, f="故障") -> (s? t:f=w1187:string)
                                }
                                n745 = Insert Into Array(array=w1175, new element=w1174) -> (w1173:string[])  [unwired: 1 in]
                              }
                              n746 = call "详细故障分解.vi"("名称"=string[] ["DI1对地短", "DI1对电源短", "DI2对地短", "DI2对电源短", "DI3对地短", "DI3对电源短", "DI4对地短", "DI4对电源短", "DI5对地短", "DI5对电源短", "DI6对地短", "DI6对电源短", "DI7对地短", "DI7对电源短", "DI8对地短", "DI8对电源短", "DO1对地短", "DO1对电源短", "DO2对地短", "DO2对电源短", "DO3对地短", "DO3对电源短", "DO4对地短", "DO4对电源短", "DO5对地短", "DO5对电源短", "DO6对地短", "DO6对电源短", "DO7对地短", "DO7对电源短", "DO8对地短", "DO8对电源短"], "故障输入口"=w1167) -> ("输出数组"=w1165:string[][])  [unwired: 1 in, 2 out]
                              n747 = local write "电池故障"(w1165) -> ()
                            }
                            frame 7 {
                              n748 = for {
                                N: 2 -> [_]
                                tunnel: w1196 -> [w1213]
                                shift-right: [w1200] -> w1194
                                shift-left: string[] [] -> [w1202]
                                i -> [w1198]
                                w1207 = 8 ("索引")
                                w1211 = 2 ("y")
                                n749 = Multiply(x=w1198, y=w1211) -> (x*y=w1212:i32)
                                n750 = Array Subset(array=w1213, index=w1212, length=w1211) -> (w1210:u8[])
                                n751 = Index Array(array=w1210) -> (element #1=w1209:u8, element #2=w1208:u8)  [unwired: 2 in]
                                n752 = call "二进制解析-8.6.vi"("索引"=w1207, "数值"=w1209) -> ("低位子数组"=w1206:i32[])  [unwired: 1 in, 2 out]
                                n753 = call "二进制解析-8.6.vi"("索引"=w1207, "数值"=w1208) -> ("低位子数组"=w1205:i32[])  [unwired: 1 in, 2 out]
                                n754 = Insert Into Array(array=w1206, new element=w1205) -> (w1204:i32[])  [unwired: 1 in]
                                n755 = case shown="1" w1198 {
                                tunnel: [4 6] -> w1199
                                frame 0, Default {
                                }
                                frame 1 {
                                }
                                }
                                n756 = Reverse 1D Array(array=w1204) -> (reversed array=w1203:i32[])
                                n757 = for {
                                N: w1199 -> [_]
                                tunnel: w1203 -> [w1220] mode=indexing
                                tunnel: [w1216] -> w1201 mode=indexing
                                n758 = Equal To 0?(x=w1220) -> (x = 0?=w1219:bool)
                                n759 = Select(t="无", s=w1219, f="故障") -> (s? t:f=w1216:string)
                                }
                                n760 = Insert Into Array(array=w1202, new element=w1201) -> (w1200:string[])  [unwired: 1 in]
                              }
                              n761 = call "详细故障分解.vi"("名称"=string[] ["超时(pre-chg)", "后端开路(pre-chg)", "后端短路(pre-chg)", "预充电回路断开(pre-chg)", "正级继电器驱动故障(relay_driver)", "负级继电器驱动故障(relay_driver)", "预充电继电器驱动故障(relay_driver)", "充电继电器驱动故障(relay_driver)", "风机继电器驱动故障(relay_driver)", "加热继电器驱动故障(relay_driver)"], "故障输入口"=w1194) -> ("输出数组"=w1192:string[][])  [unwired: 1 in, 2 out]
                              n762 = local write "电池故障"(w1192) -> ()
                            }
                          }
                        }
                        frame True {
                          n763 = Index Array(array=w1224, index #1=0 ("索引"), index #2=1 ("索引")) -> (element #1=w1227:u8, element #2=w1228:u8)
                          n764 = Join Numbers(hi=w1227, lo=w1228) -> ((hi.lo)=w1226:u16)
                          n765 = Number To Hexadecimal String(2:w1226) -> (0:w1225:string)  [unwired: 1 out]
